vi "OBJ_initialize_manual_editors.vi"(8 "error_in":errorcluster, 11 "all_config_info":T1={"main_ini_file"={"SQL Driver"="", "SQL Server"="", "SQL Database"="", "SQL UID"="", "User table"="", "Reference table"="", "default language"="", "SCANNER COM port"=0, "SCANNER Baud rate"=0, "SCANNER Data bits"=0, "SCANNER Pairity"=enum."None", "SCANNER Stop bits"=0, "SCANNER Flow control"=0, "SCANNER Termination char"=0, "MD-L COM port"=0, "MD-L Baud rate"=10, "MD-L Data bits"=0, "MD-L Pairity"=enum."None", "MD-L Stop bits"=0, "MD-L Flow control"=0, "MD-L Termination char"=0, "MD-R COM port"=0, "MD-R Baud rate"=0, "MD-R Data bits"=0, "MD-R Pairity"=enum."None", "MD-R Stop bits"=10, "MD-R Flow control"=0, "MD-R Termination char"=0, "logout timeout [ms]"=0}, "SQL Password"="", "queue_refnums"={"MAIN_queue"=refnum, "SCANNER_queue"=refnum, "SCANNER_login"=refnum, "MD_L_queue"=refnum, "MD_L_data"=refnum, "MD_R_queue"=refnum, "MD_R_data"=refnum, "OBJ_GUI_TIMER_queue"=refnum}} {"main_ini_file"."MD-R Flow control" items=["None"=0, "XON/XOFF"=1, "RTS/CTS"=2, "DTR/DSR"=4]; "main_ini_file"."MD-R Stop bits" items=["1.0"=10, "1.5"=15, "2.0"=20]; "main_ini_file"."MD-L Flow control" items=["None"=0, "XON/XOFF"=1, "RTS/CTS"=2, "DTR/DSR"=4]; "main_ini_file"."MD-L Stop bits" items=["1.0"=10, "1.5"=15, "2.0"=20]; "main_ini_file"."SCANNER Flow control" items=["None"=0, "XON/XOFF"=1, "RTS/CTS"=2, "DTR/DSR"=4]; "main_ini_file"."SCANNER Stop bits" items=["1.0"=10, "1.5"=15, "2.0"=20]}) -> (0 "error_out":errorcluster)   [LabVIEW 2019]
uses:
  ini/typedef/OBJ_all_config_info.ctl
  ini/typedef/OBJ_main_ini_file.ctl
  queues/typedef/OBJ_queue_refnums.ctl
  queues/typedef/OBJ_MAIN_queue_element.ctl
  MAIN/OBJ_MAIN_sequence_state.ctl
  queues/typedef/OBJ_SCANNER_queue_element.ctl
  SCANNER/OBJ_SCANNER_sequence_state.ctl
  queues/typedef/OBJ_MD_queue_element.ctl
  MEASURING_DEVICE/OBJ_MD_sequence_state.ctl
  queues/typedef/OBJ_GUI_TIMER_queue_element.ctl
  GUI_TIMER/OBJ_GUI_TIMER_sequence_state.ctl
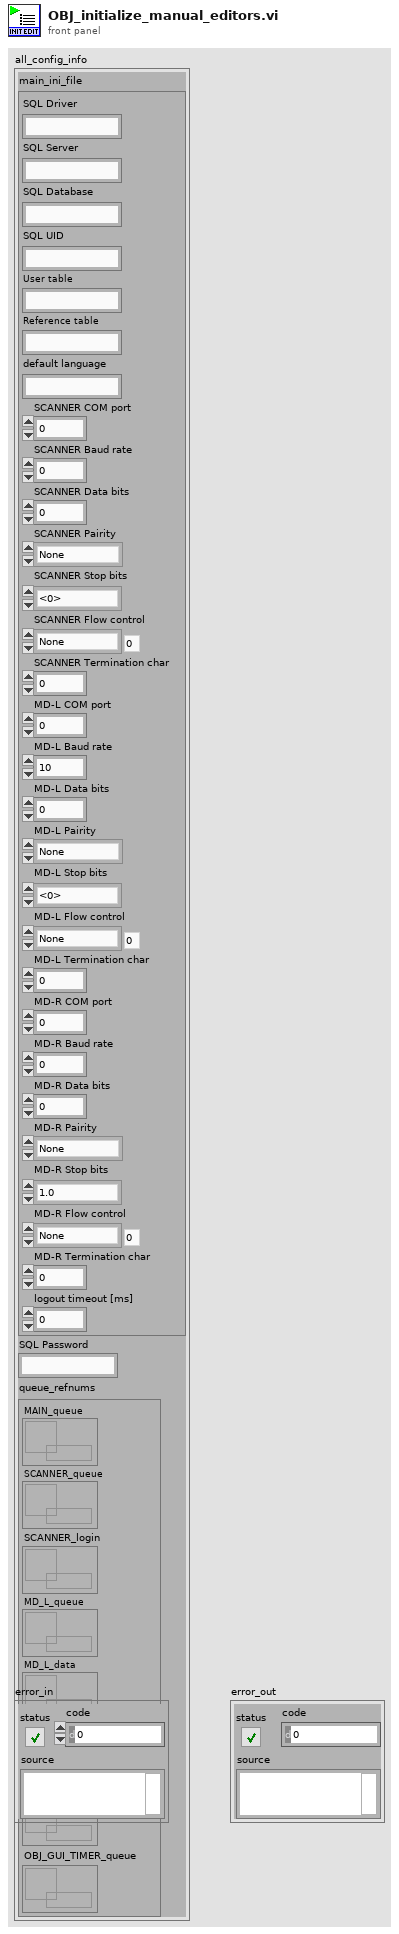
[diagram p1: front panel]
types:
  T1 = typedef "OBJ_all_config_info.ctl" = cluster{"main_ini_file":T2, "SQL Password":string, "queue_refnums":T3}
  T2 = typedef "OBJ_main_ini_file.ctl" = cluster{"SQL Driver":string, "SQL Server":string, "SQL Database":string, "SQL UID":string, "User table":string, "Reference table":string, "default language":string, "SCANNER COM port":u16, "SCANNER Baud rate":u32, "SCANNER Data bits":u16, "SCANNER Pairity":enum16{"None", "Odd", "Even", "Mark", "Space"}, "SCANNER Stop bits":u16, "SCANNER Flow control":u16, "SCANNER Termination char":u8, "MD-L COM port":u16, "MD-L Baud rate":u32, "MD-L Data bits":u16, "MD-L Pairity":enum16{"None", "Odd", "Even", "Mark", "Space"}, "MD-L Stop bits":u16, "MD-L Flow control":u16, "MD-L Termination char":u8, "MD-R COM port":u16, "MD-R Baud rate":u32, "MD-R Data bits":u16, "MD-R Pairity":enum16{"None", "Odd", "Even", "Mark", "Space"}, "MD-R Stop bits":u16, "MD-R Flow control":u16, "MD-R Termination char":u8, "logout timeout [ms]":i32}
  T3 = typedef "OBJ_queue_refnums.ctl" = cluster{"MAIN_queue":refnum<queue>, "SCANNER_queue":refnum<queue>, "SCANNER_login":refnum<queue>, "MD_L_queue":refnum<queue>, "MD_L_data":refnum<queue>, "MD_R_queue":refnum<queue>, "MD_R_data":refnum<queue>, "OBJ_GUI_TIMER_queue":refnum<queue>}
  T4 = typedef "OBJ_MAIN_queue_element.ctl" = cluster{"state":T5, "variable":variant}
  T5 = typedef "OBJ_MAIN_sequence_state.ctl" = enum16{"initialize", "get_next_state", "read_reference_list", "USER_login", "USER_logout", "read_gear_data", "perform_test", "start_timer", "clear_test_data", "error", "stop"}
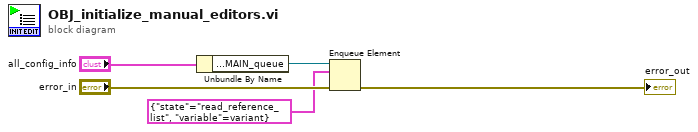
[diagram p0: block diagram]
diagram:
  n1 = Unbundle By Name("all_config_info") -> ("queue_refnums.MAIN_queue"=w5:refnum<queue>)
  n2 = Enqueue Element(queue=w5, element=T4 {"state"=enum."read_reference_list", "variable"=variant}, error in (no error)="error_in") -> (error out=→"error_out":errorcluster)  [unwired: 1 in, 2 out]
